vi "hostToFPGA(Array).vi"(7 "Write Timeout (ms)":i32=5000, 8 "error in (no error)":errorcluster, 9 "Image in":T1, 10 "Maximum Pixels per Write":i32=-1, 11 "Refnum in":refnum<k20>) -> (0 "error out":errorcluster, 2 "Image Out":T1, 3 "Refnum out":refnum<k20>)   [LabVIEW 2016]
uses:
  <vilib>/vision/Image Controls.llb/IMAQ Image.ctl
  <vilib>/vision/EDVR.llb/IMAQ ImageToEDVR 2D U32.vi
  <vilib>/rvi/errors/niLvFpgaAdjustHostInterfaceError.vi
  <vilib>/rvi/interface/nirviMethod/nirviMethod.xnode
  <vilib>/FPGAPlugInAG/Dynamic/niLvFpga_WriteFifo_Dynamic.vi
  <vilib>/rvi/errors/niLvFpgaMergeErrorWithErrorCode.vi
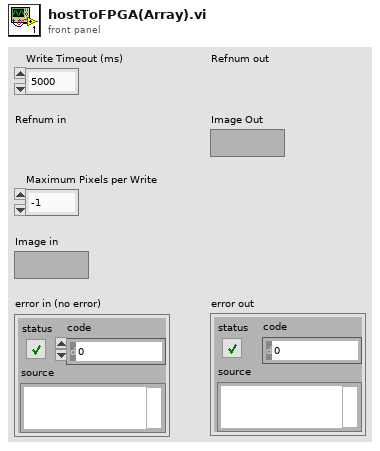
[diagram p1: front panel]
types:
  T1 = typedef "IMAQ Image.ctl" = refnum<image>
  T2 = typedef "Image Type" = u32
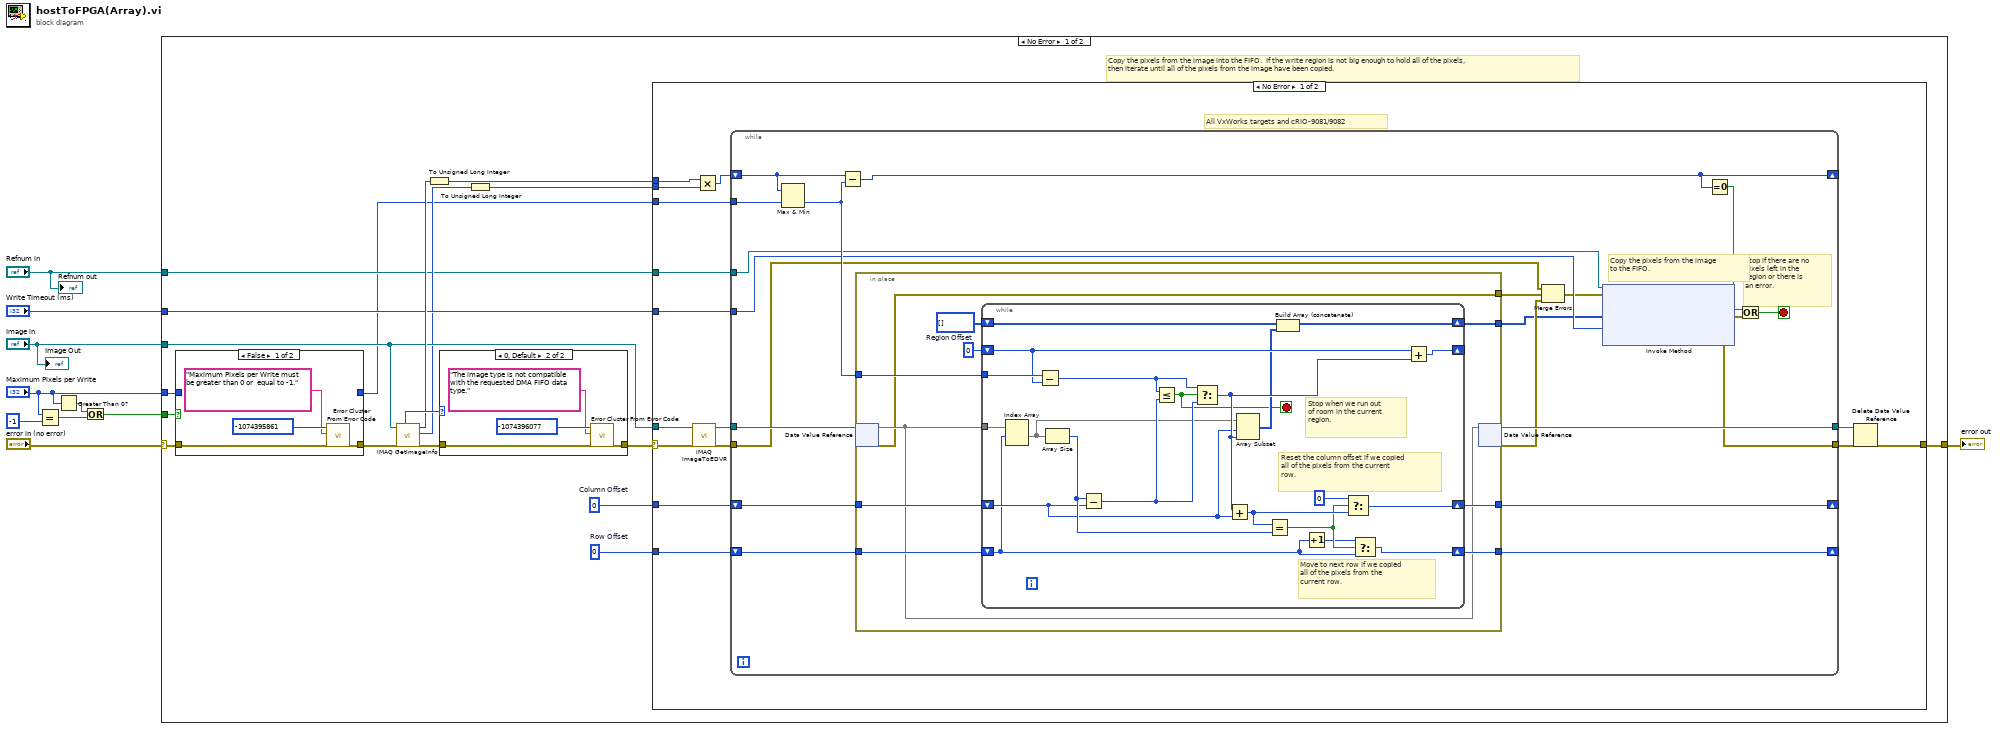
[diagram p0: block diagram]
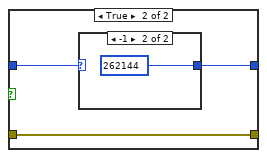
[diagram p3: hidden frame]
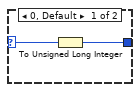
[diagram p4: hidden frame]
diagram:
  n1 = Equal?(x="Maximum Pixels per Write", y=-1) -> (x = y?=w5:bool)
  n2 = Greater Than 0?(x="Maximum Pixels per Write") -> (x > 0?=w4:bool)
  n3 = Or(x=w4, y=w5) -> (x .or. y?=w6:bool)
  n4 = case shown="No Error" "error in (no error)" {
    selector: "error in (no error)" -> [w23 w111]
    tunnel: "Refnum in" -> [w14 _]
    tunnel: "Write Timeout (ms)" -> [w16 _]
    tunnel: w6 -> [w26 _]
    tunnel: "Maximum Pixels per Write" -> [w24 _]
    tunnel: "Image in" -> [w18 _]
    tunnel: [w21 w111] -> w9
    frame No Error {
      w20 = u32 0  # Row Offset
      w19 = u32 0  # Column Offset
      # "Copy the pixels from the image into the FIFO.  If the write region is not big enough to hold all of the pixels,\nthen iterate until all of the pixels from the image have been copied."
      n5 = case shown="False" w26 {
        tunnel: w23 -> [w97 w102]
        tunnel: [w96 w102] -> w25
        tunnel: w24 -> [_ w101]
        tunnel: [_ w100] -> w13
        frame False {
          n6 = call <vilib>:"Error Cluster From Error Code.vi"("error in (no error)"=w97, "error message (\"\")"="Maximum Pixels per Write must be greater than 0 or  equal to -1." ("error message (\"\")"), "error code (0)"=-1074395861) -> ("error out"=w96:errorcluster)  [unwired: 6 in]
        }
        frame True {
          n7 = case shown="-1" w101 {
            selector: w101 -> [w104 _]
            tunnel: [w103 u32 262144 ("Maximum Pixels per Write")] -> w100
            frame 0, Default {
              n8 = To Unsigned Long Integer(number=w104) -> (unsigned 32bit integer=w103:u32)
            }
            frame -1 {
            }
          }
        }
      }
      n9 = call "IMAQ GetImageInfo"("error in (no error)"=w25, "Image"=w18) -> ("error out"=w27:errorcluster, "Y Resolution"=w15:i32, "X Resolution"=w22:i32, "Image Type"=w28:T2)  [unwired: 2 in, 4 out]
      n10 = To Unsigned Long Integer(number=w22) -> (unsigned 32bit integer=w12:u32)
      n11 = case shown="0, Default" w28 {
        tunnel: w27 -> [w106 w108]
        tunnel: [w106 w107] -> w17
        frame 4, 5 {
          # "Allowed types are:\nRGB (U32)\nHSL (U32)"
        }
        frame 0, Default {
          n12 = call <vilib>:"Error Cluster From Error Code.vi"("error in (no error)"=w108, "error message (\"\")"="The image type is not compatible with the requested DMA FIFO data type." ("error message (\"\")"), "error code (0)"=-1074396077) -> ("error out"=w107:errorcluster)  [unwired: 6 in]
        }
      }
      n13 = To Unsigned Long Integer(number=w15) -> (unsigned 32bit integer=w11:u32)
      n14 = case shown="No Error" w17 {
        selector: w17 -> [w38 w95]
        tunnel: w19 -> [w40 _]
        tunnel: w20 -> [w39 _]
        tunnel: w14 -> [w42 _]
        tunnel: [w36 w95] -> w21
        tunnel: w13 -> [w43 _]
        tunnel: w16 -> [w41 _]
        tunnel: w18 -> [w37 _]
        tunnel: w12 -> [w35 _]
        tunnel: w11 -> [w34 _]
        frame No Error {
          # "All VxWorks targets and cRIO-9081/9082"
          n15 = call-poly <vilib>:"IMAQ ImageToEDVR.vi"("error out"=w38, "Image"=w37) -> ("error out"=w32:errorcluster, "EDVR 2D U32"=w33:refnum<data-value>)  [unwired: 7 in, 1 out]
          n16 = Multiply(x=w35, y=w34) -> (x*y=w29:u32)
          n17 = while {
            shift-right: [w57] -> _
            shift-left: w29 -> [w54]
            tunnel: w33 -> [w63]
            shift-right: [w59] -> _
            shift-left: w40 -> [w61]
            shift-right: [w62] -> _
            shift-left: w39 -> [w60]
            tunnel: w42 -> [w48]
            tunnel: [w58] -> w31
            tunnel: [w46] -> w30
            tunnel: w43 -> [w53]
            tunnel: w41 -> [w49]
            tunnel: w32 -> [w44]
            stop <- w56 stop-if-true
            # "Copy the pixels from the image\nto the FIFO."
            # "Stop if there are no\npixels left in the \nregion or there is\nan error."
            n18 = Max & Min(x=w54, y=w53) -> (min(x,y)=w52:u32)  [unwired: 1 out]
            n19 = Subtract(x=w54, y=w52) -> (x-y=w57:u32)
            n20 = in-place {
              in-place-border: w52 -> [w71]
              in-place-border: [w73] -> w62
              in-place-border: w61 -> [w70]
              in-place-border: w60 -> [w68]
              in-place-border: [w69] -> w59
              in-place-border: [w65] -> w51
              in-place-border: [w64] -> w45
              w72 = u32 0  # Region Offset
              n21 = in-place-dvr #1(w63) -> (w67:u32[][], w65:errorcluster)
              n22 = while {
                tunnel: w67 -> [w80]
                shift-right: [w92] -> _
                shift-left: w72 -> [w91]
                tunnel: w71 -> [w94]
                shift-right: [w85] -> w69
                shift-left: w70 -> [w81]
                shift-right: [w75] -> w64
                shift-left: u8[] [] -> [w77]
                shift-right: [w82] -> w73
                shift-left: w68 -> [w78]
                stop <- w74 stop-if-true
                # "Stop when we run out\nof room in the current\nregion."
                # "Reset the column offset if we copied\nall of the pixels from the current\nrow."
                # "Move to next row if we copied\nall of the pixels from the\ncurrent row."
                n23 = Index Array(array=w80, index (row)=w78) -> (element=w79:u32[])  [unwired: 1 in]
                n24 = Subtract(x=w94, y=w91) -> (x-y=w93:u32)
                n25 = Array Size(array=w79) -> (size(s)=w90:i32)
                n26 = Subtract(x=w90, y=w81) -> (x-y=w88:u32)
                n27 = Less Or Equal?(x=w93, y=w88) -> (x <= y?=w74:bool)
                n28 = Select(t=w93, s=w74, f=w88) -> (s? t:f=w89:u32)
                n29 = Add(x=w89, y=w81) -> (x+y=w86:u32)
                n30 = Array Subset(array=w79, index=w81, length=w89) -> (w76:u32[])
                n31 = Equal?(x=w86, y=w90) -> (x = y?=w84:bool)
                n32 = Build Array (concatenate)(w77, w76) -> (w75:u32[])
                n33 = Increment(x=w78) -> (x+1=w83:u32)
                n34 = Select(t=u32 0 ("Elements In Region"), s=w84, f=w86) -> (s? t:f=w85:u32)
                n35 = Select(t=w83, s=w84, f=w78) -> (s? t:f=w82:u32)
                n36 = Add(x=w91, y=w89) -> (x+y=w92:u32)
              }
              n37 = in-place-dvr #1(w67) -> (w58:refnum<data-value>, w50:errorcluster)
            }
            n38 = Merge Errors(w44, w51, w50) -> (w47:errorcluster)
            n39 = xnode "Invoke Method"("FPGA VI Reference In"=w48, "error in"=w47, "Data"=w45, "Timeout (ms)"=w49) -> ("error out"=w46:errorcluster)  [unwired: 2 out]
            n40 = Equal To 0?(x=w57) -> (x = 0?=w55:bool)
            n41 = Or(x=w55, y=w46) -> (x .or. y?=w56:bool)
          }
          n42 = Delete Data Value Reference(data value reference=w31, error in=w30) -> (error out=w36:errorcluster)  [unwired: 1 out]
        }
        frame Error {
        }
      }
    }
    frame Error {
    }
  }
  "error out" <- w9
  "Image Out" <- "Image in"
  "Refnum out" <- "Refnum in"
